vi "HRM-common-Status_feedback.vi"(7 "Module name":string, 8 "error in (no error)":errorcluster, 11 "init cluster":T1) -> (0 "error out":errorcluster)   [LabVIEW 2020]
uses:
  HRM-init-cluster.ctl
  HRM-init-user_events.ctl
  process/HRM-process-Pulse settings.ctl
  HRM-init-Intial State.ctl
  HRM-init-hardware_selector.ctl
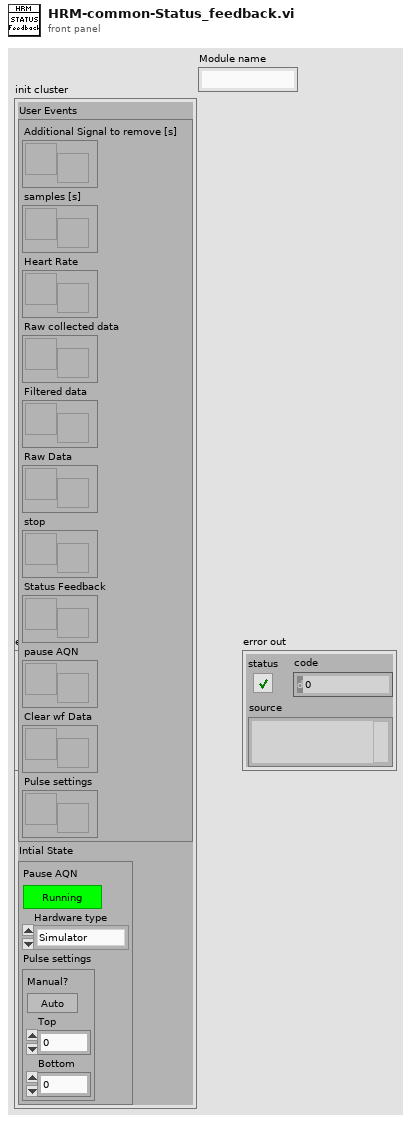
[diagram p1: front panel]
types:
  T1 = typedef "HRM-init-cluster.ctl" = cluster{"User Events":T2, "Intial State":T3}
  T2 = typedef "HRM-init-user_events.ctl" = cluster{"Additional Signal to remove [s]":refnum<user-event>, "samples [s]":refnum<user-event>, "Heart Rate":refnum<user-event>, "Raw collected data":refnum<user-event>, "Filtered data":refnum<user-event>, "Raw Data":refnum<user-event>, "stop":refnum<user-event>, "Status Feedback":refnum<user-event>, "pause AQN":refnum<user-event>, "Clear wf Data":refnum<user-event>, "Pulse settings":refnum<user-event>}
  T3 = typedef "HRM-init-Intial State.ctl" = cluster{"Pause AQN":bool, "Hardware type":T4, "Pulse settings":T5}
  T4 = typedef "HRM-init-hardware_selector.ctl" = enum16{"Simulator", "myDAQ", "Arduino", "Analog Discovery"}
  T5 = typedef "HRM-process-Pulse settings.ctl" = cluster{"Manual?":bool, "Top":dbl, "Bottom":dbl}
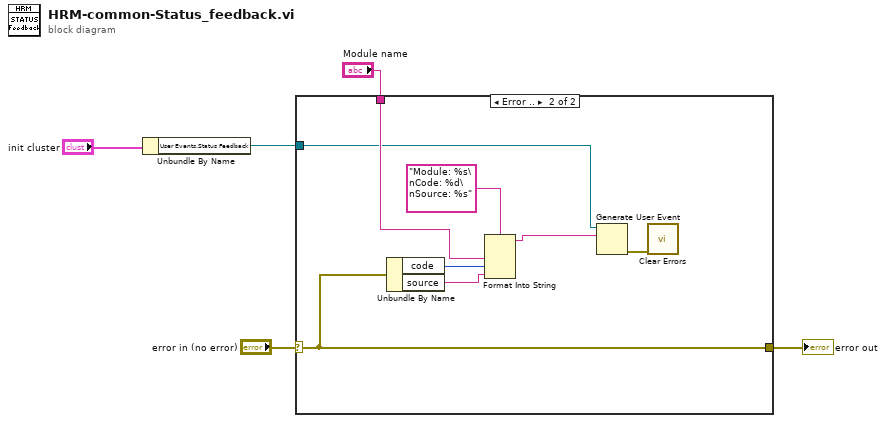
[diagram p0: block diagram]
diagram:
  n1 = Unbundle By Name("init cluster") -> ("User Events.Status Feedback"=w1:refnum<user-event>)
  n2 = case shown="Error .." "error in (no error)" {
    selector: "error in (no error)" -> [w6 w14]
    tunnel: [w6 w14] -> w3
    tunnel: "Module name" -> [_ w9]
    tunnel: w1 -> [_ w7]
    frame No Error {
    }
    frame Error {
      n3 = Unbundle By Name(w14) -> ("code"=w11:i32, "source"=w10:string)
      n4 = Format Into String(format string="Module: %s\nCode: %d\nSource: %s", w9, w11, w10) -> (resulting string=w8:string)  [unwired: 2 in, 1 out]
      n5 = Generate User Event(user event=w7, event data cluster=w8) -> (error out=w13:errorcluster)  [unwired: 2 in, 1 out]
      n6 = call <vilib>:"Clear Errors.vi"("error in (no error)"=w13) -> ()  [unwired: 5 in, 2 out]
    }
  }
  "error out" <- w3
